vi "Centrifuge Module (Main).vi"(7 "Name of Parent Panel":string="Main.vi", 9 "New Center Coords":T1={"Horizontal"=470, "Vertical"=200}, 10 "Config":variant, 11 "Main UI Message Queue":refnum<queue>) -> ()   [LabVIEW 2018, in "Centrifuge Module.lvlib"]
doc: "This Continuous Measurement sample project is based on the Queued Message Handler template.\n\nThe Event Handling Loop generates messages based on user interface actions.\n\nThe Message Handling Loop processes messages generated by the Event Handling Loop, or by other messages. There are also Acquisition and Logging message handling loop subVIs, and a chart updating loop."
uses:
  Centrifuge Module.lvlib
  support/Message Queue/Message Cluster.ctl
  <vilib>/Utility/miscctls.llb/LVPoint32TypeDef.ctl
  controls/UI Data.ctl
  controls/UI State.ctl
  Centrifuge Module State Cluster.ctl
  Centrifuge Module Config Cluster.ctl
  Centrifuge Module Settings Cluster.ctl
  EPOS4/Controls/Device Selection.ctl
  EPOS4/Controls/EPOS Communication Settings.ctl
  Measure Instrument/State Enum.ctl
  Sequencing/Squence Update Cluster.ctl
  Centrifuge Module Display.ctl
  support/Message Queue/Enqueue Message (Single).vi
  support/User Event - Stop/User Event - Stop.lvlib
  support/Support Library.lvlib
  support/Message Queue/Message Queue.lvlib
  Measure Instrument/Centrifuge Module Engine.lvlib
  Measure Instrument/Feed Module Engine.lvlib
  Sequencing/Sequencing Library.lvlib
  Centrifuge Settings Dialog.vi
  support/Command Log VIs/Command Logging.lvlib
  EPOS4/EPOS4.lvlib
panel:
  out "Display Cluster":cluster{"User Name":string, "Speed":dbl} {"Speed" format="%#_5g"}
  out "H/W":dbl
  out "Original Height":u32
  out "Original Width":u32
  in  "Settings Button":bool
  out "Sequence Started":bool
  out "ScanCode":i16
  out "Ring":u16(ring)=2
  out "Log File path":path
  out "Status":string
  in  "Exit":bool
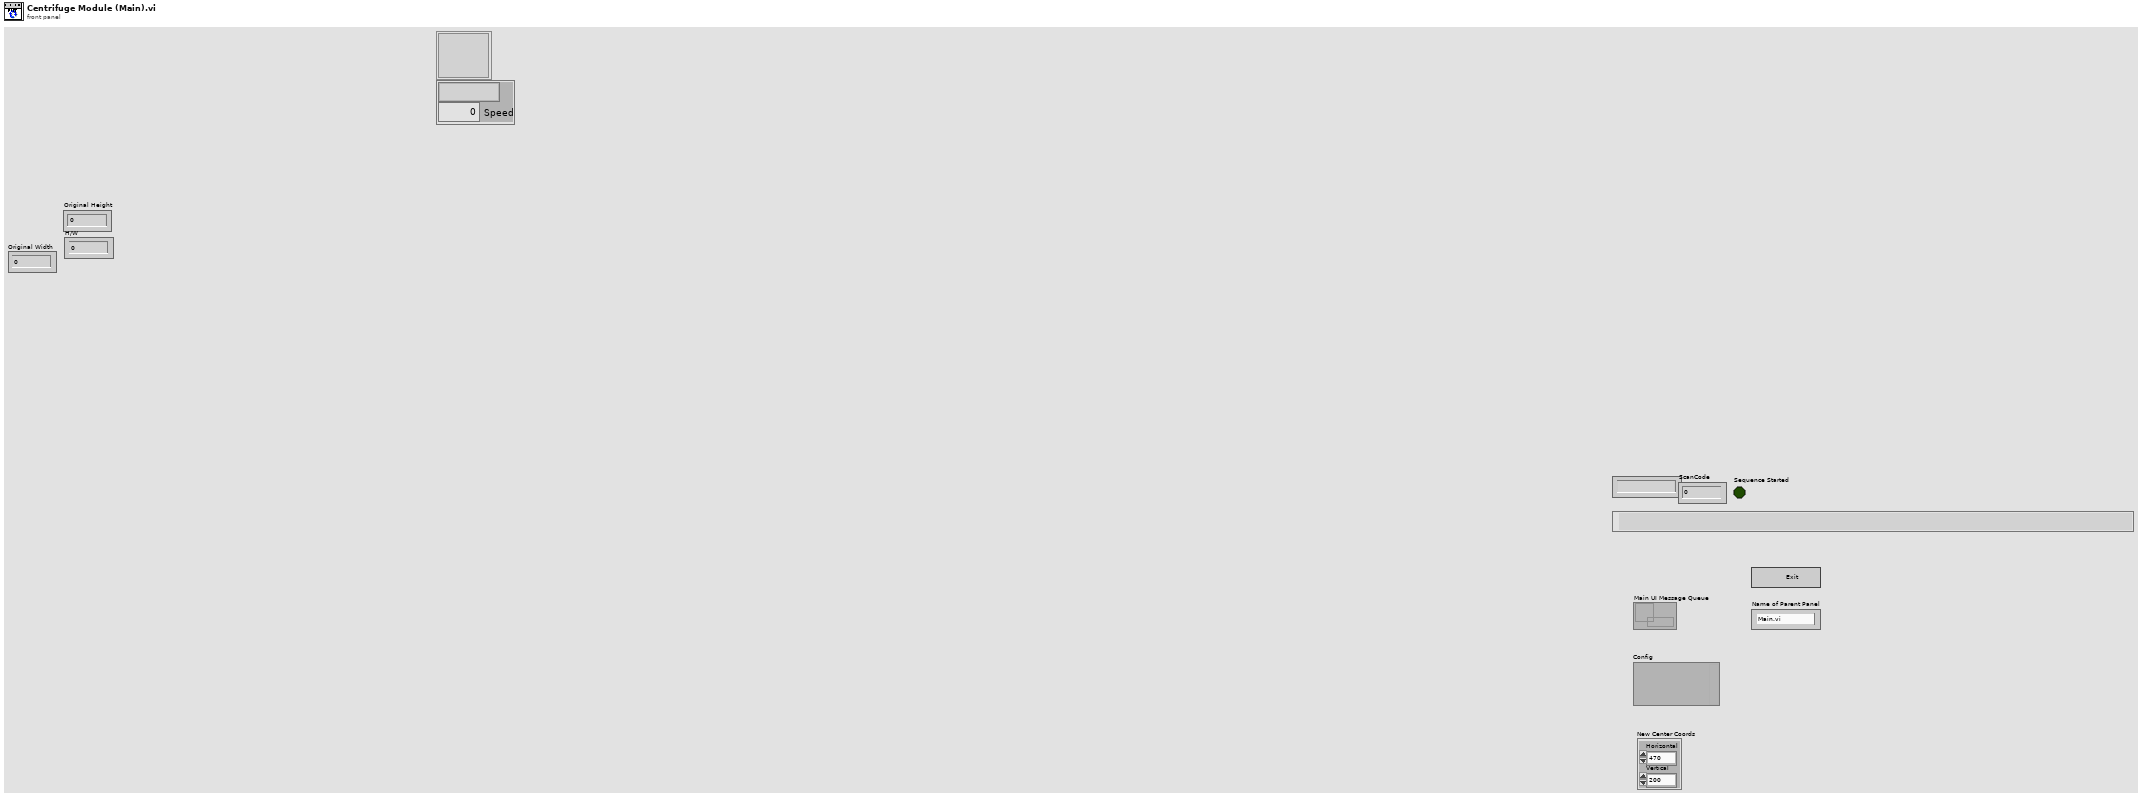
[diagram p1: front panel]
types:
  T1 = typedef "LVPoint32TypeDef.ctl" = cluster{"Horizontal":i32, "Vertical":i32}
  T2 = enum32{"Invalid", "Default", "Floating", "Floating/Auto-Hide", "Modal"}
  T3 = typedef "UI State.ctl" = enum16{"Idle", "Acquiring and Logging", "Waiting for Exit", "Waiting for Exit (Acq Stopped)", "Waiting for Exit (Log Stopped)", "Waiting for Stop", "Waiting for Stop (Acq Stopped)", "Waiting for Stop (Log Stopped)"}
  T4 = typedef "UI Data.ctl" = cluster{"Start Ref":refnum<vi>, "Trigger Ref":refnum<vi>, "Stop Ref":refnum<vi>, "Settings Ref":refnum<vi>, "Status Ref":refnum<vi>, "Exit Ref":refnum<vi>, "Data Ref":refnum<vi>}
  T5 = typedef "Centrifuge Module.lvlib/Centrifuge Module Config Cluster.ctl" = cluster{"GUID":string, "Drop Coords":T1, "Process Name":string, "User name":string, "Queue Name":string, "Settings":T6, "Load Count":i32}
  T6 = typedef "Centrifuge Module.lvlib/Centrifuge Module Settings Cluster.ctl" = cluster{"Cycle Period":dbl, "Manual Entry":dbl, "Output Device":T7, "EPOS4 Settings":T8}
  T7 = typedef "Device Selection.ctl" = enum16{"Default", "EPOS4"}
  T8 = typedef "EPOS4.lvlib/EPOS Communication Settings.ctl" = cluster{"VISA resource name":refnum<visa-resource-name>, "axis":cluster{"keyHandle":u32, "nodeId":u16}, "Simulated?":bool}
  T9 = typedef "Centrifuge Module.lvlib/Centrifuge Module State Cluster.ctl" = cluster{"Centrifuge Module Config":T5, "State":T10, "Start Time":timestamp, "Current Time":timestamp, "First Iteration":bool, "Data":cluster{"Centrifuge Speed":dbl}, "Process Name":string, "Centrifuge On?":bool}
  T10 = typedef "Feed Module.lvlib/Feed Module Engine.lvlib/State Enum.ctl" = enum16{"Measuring", "Idle", "Paused"}
  T11 = typedef "LVPointTypeDef.ctl" = cluster{"Horizontal":i16, "Vertical":i16}
  T12 = typedef "Centrifuge Module.lvlib/All Message Queues.ctl" = cluster{"Engine":refnum<queue>, "Centrifuge UI":refnum<queue>, "Centrifuge Engine":refnum<queue>, "Centrifuge Display":refnum<queue>}
  T13 = typedef "Sequencing Library.lvlib/Squence Update Cluster.ctl" = cluster{"Auto?":bool, "Manual Entry":dbl, "Setpoint":dbl}
  T14 = enum8{"Enabled", "Disabled", "Disabled and Grayed Out"}
  T15 = typedef "Centrifuge Module.lvlib/Centrifuge Module Display.ctl" = cluster{"Centrifuge On?":enum16{"Off", "On", "Not Initialized"}, "Cycle Period":dbl, "Current Centrifuge Speed":dbl, "Output":T7}
  T16 = typedef "LVRectTypeDef.ctl" = cluster{"Left":i16, "Top":i16, "Right":i16, "Bottom":i16}
  T17 = cluster{"Shift":bool, "Ctrl":bool, "Alt":bool, "Cmd":bool, "Opt":bool}
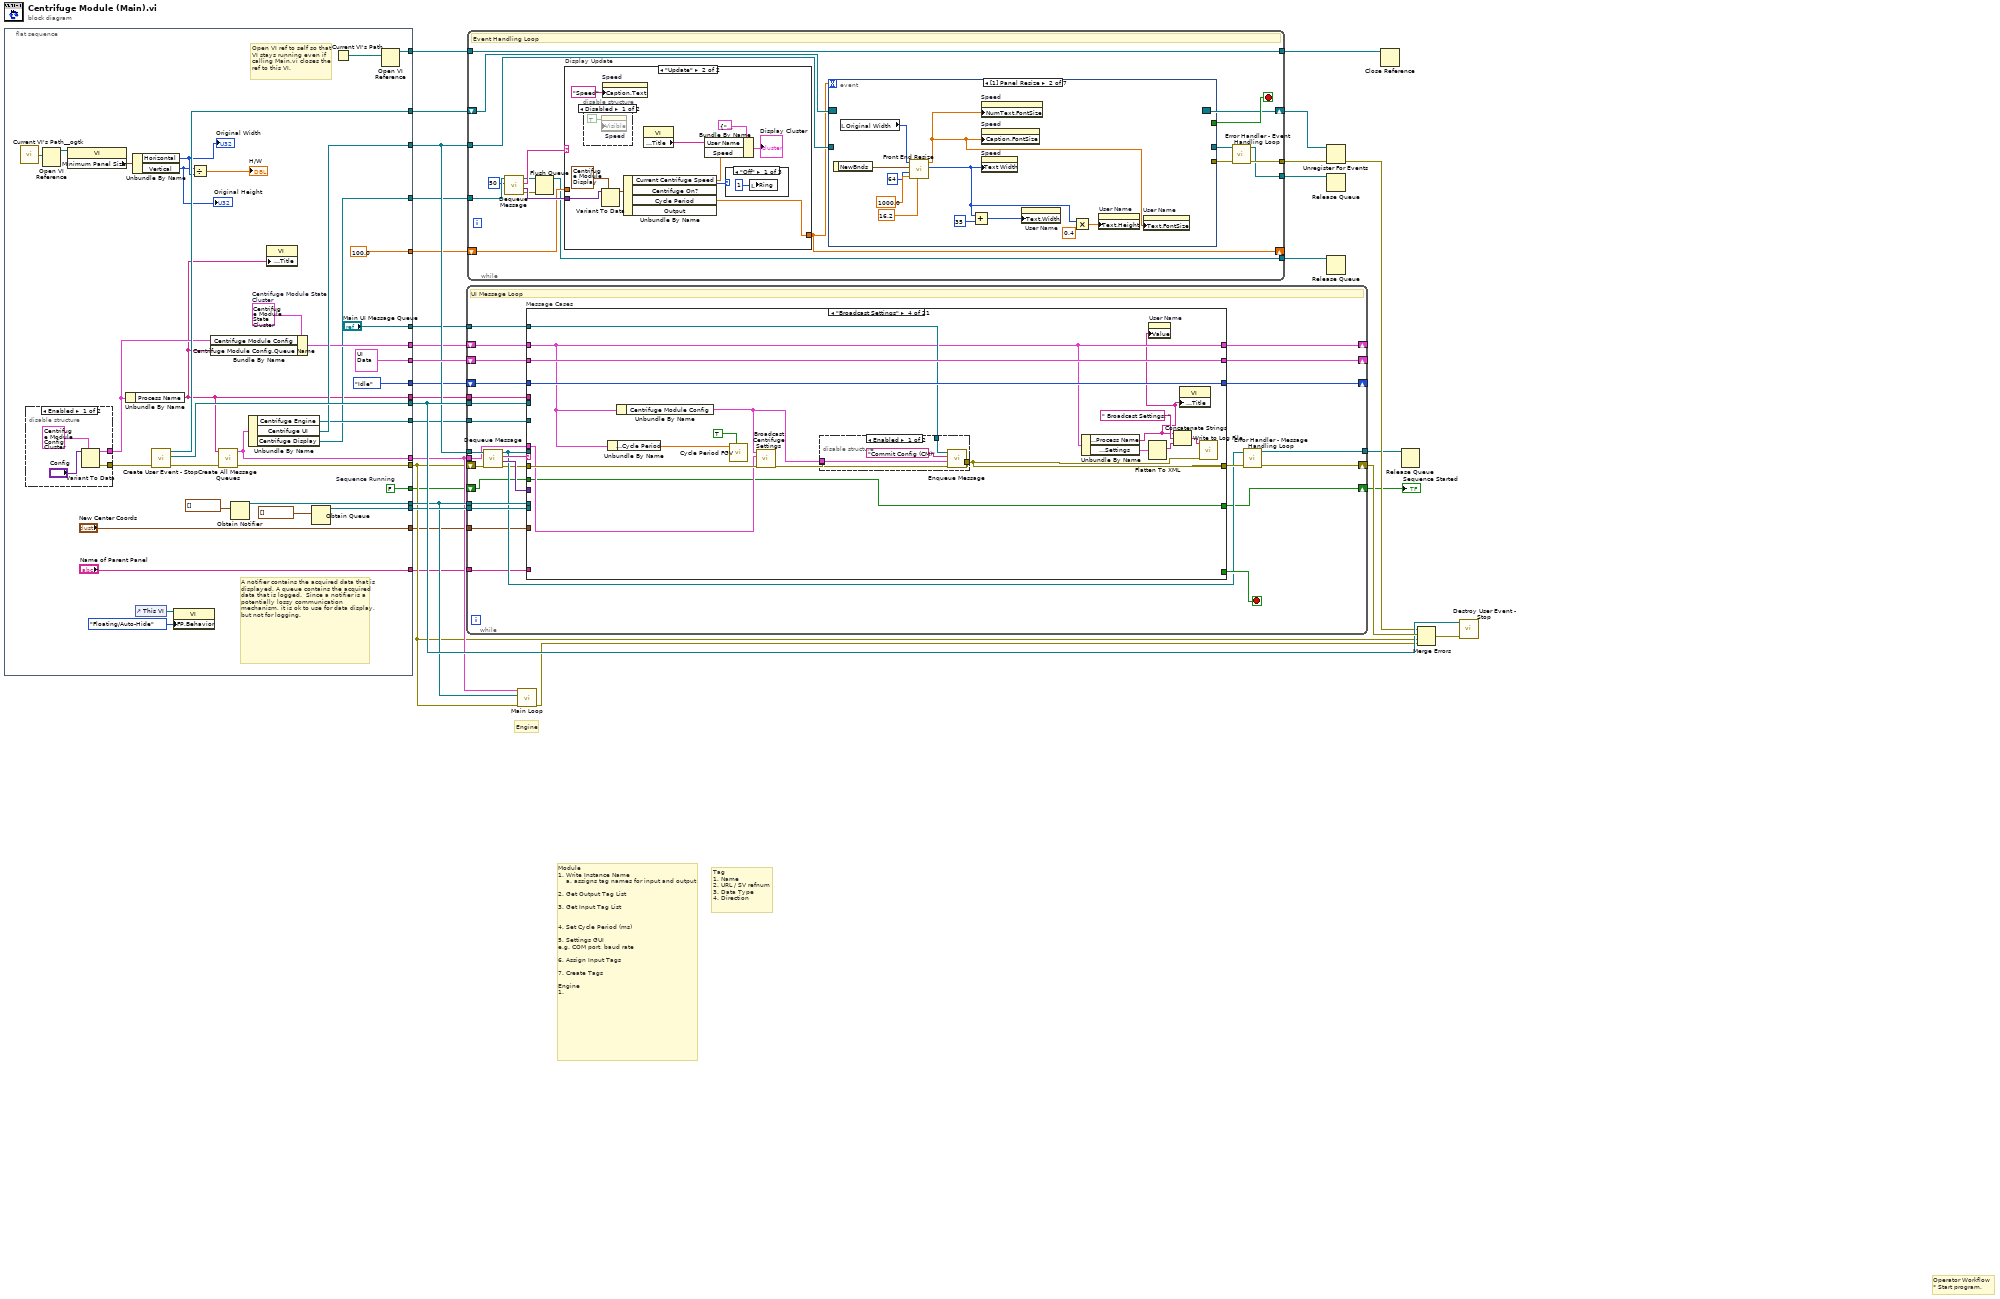
[diagram p0: block diagram]
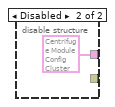
[diagram p2: hidden frame]
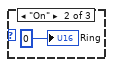
[diagram p5: hidden frame]
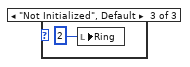
[diagram p6: hidden frame]
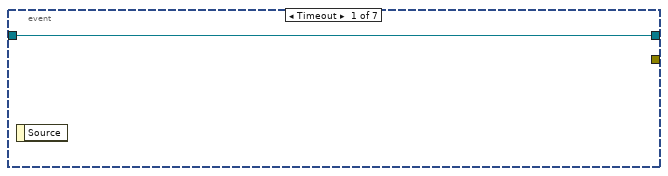
[diagram p7: hidden frame]
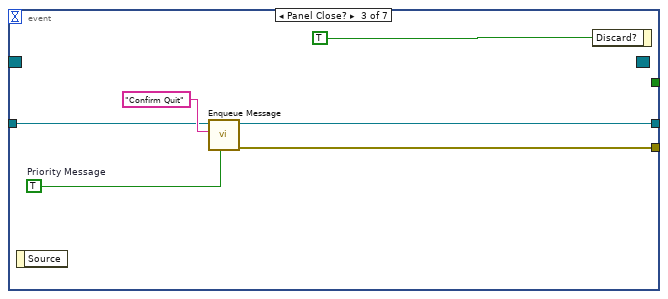
[diagram p8: hidden frame]
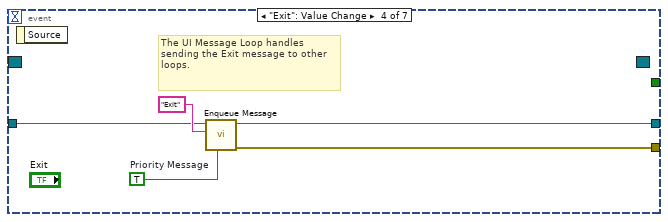
[diagram p9: hidden frame]
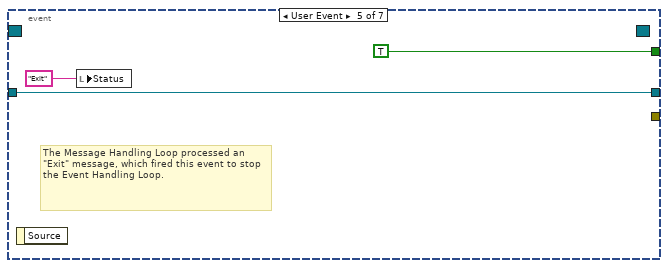
[diagram p10: hidden frame]
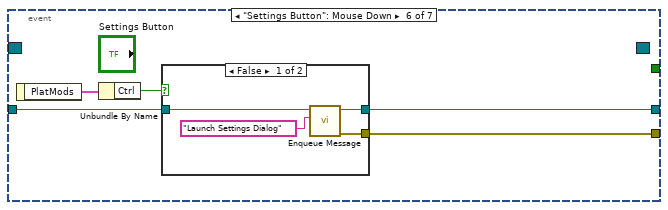
[diagram p11: hidden frame]
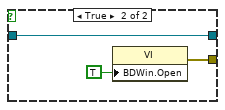
[diagram p12: hidden frame]
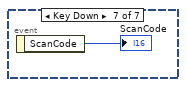
[diagram p13: hidden frame]
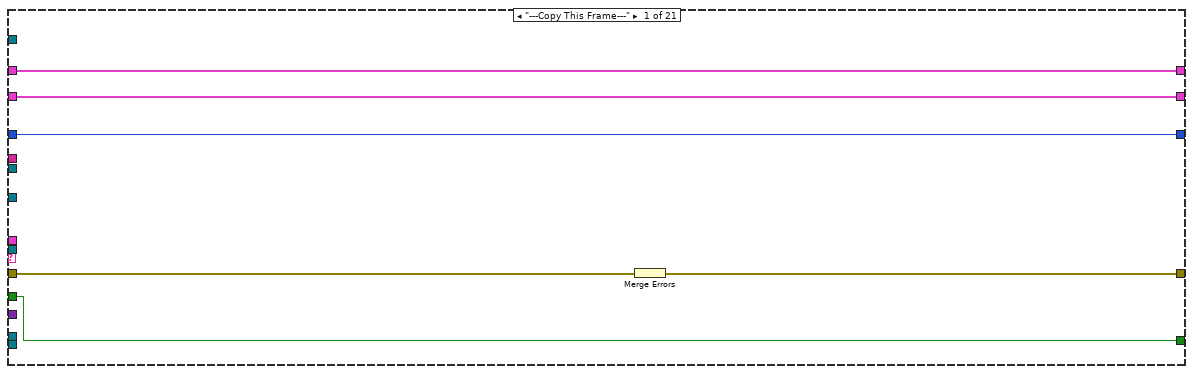
[diagram p14: hidden frame]
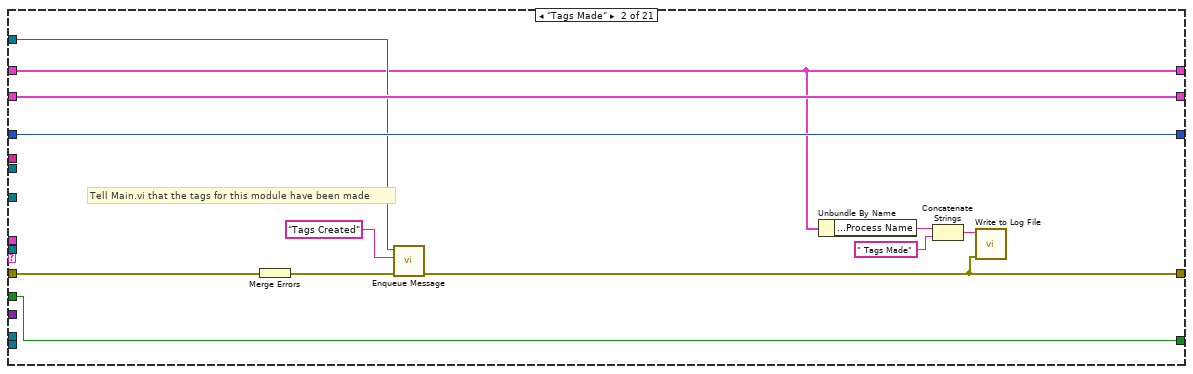
[diagram p15: hidden frame]
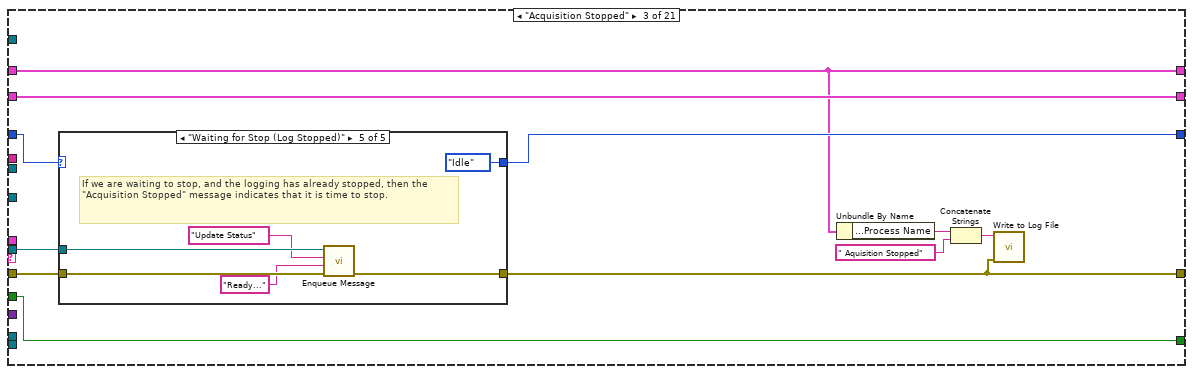
[diagram p16: hidden frame]
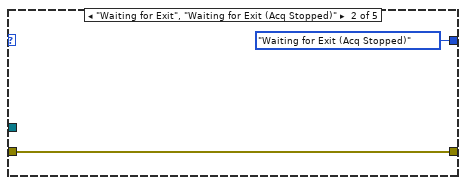
[diagram p18: hidden frame]
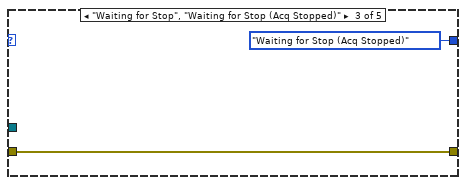
[diagram p19: hidden frame]
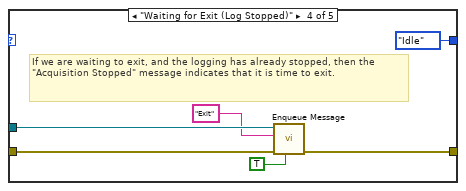
[diagram p20: hidden frame]
diagram:
  # "Engine"
  # "Operator Workflow\n* Start program."
  # "Module \n1. Write Instance Name\n    a. assigns tag names for input and output\n\n2. Get Output Tag List\n\n3. Get Input Tag List\n\n\n4. Set Cycle Period (ms)\n\n5. Settings GUI\ne.g. COM port, baud rate\n\n6. Assign Input Tags\n\n7. Create Tags\n\nEngine\n1."
  # "Tag\n1. Name\n2. URL / SV refnum\n3. Data Type\n4. Direction"
  n1 = flat-sequence {
    tunnel: [w64] -> w27
    tunnel: [w63] -> w26
    tunnel: [T4 {"Start Ref"=refnum, "Trigger Ref"=refnum, "Stop Ref"=refnum, "Settings Ref"=refnum, "Status Ref"=refnum, "Exit Ref"=refnum, "Data Ref"=refnum} ("Measurement UI Controls")] -> w23
    tunnel: [w61] -> w22
    tunnel: [UI_State."Idle" ("UI State")] -> w21
    tunnel: [w57] -> w20
    tunnel: [w56] -> w19
    tunnel: [w55] -> w17
    tunnel: [w54] -> w15
    tunnel: [w52] -> w14
    tunnel: ["Main UI Message Queue"] -> w13
    tunnel: [w47] -> w12
    tunnel: [w45] -> w11
    tunnel: [w44] -> w10
    tunnel: ["New Center Coords"] -> w9
    tunnel: ["Name of Parent Panel"] -> w8
    tunnel: [w41] -> w6
    tunnel: [w37] -> w5
    tunnel: [100.0 ("Cycle Period")] -> w4
    frame #0 {
      w41 = FALSE  # Sequence Running
      w48 = T9 {"Centrifuge Module Config"={"GUID"="", "Drop Coords"={"Horizontal"=0, "Vertical"=0}, "Process Name"="", "User name"="", "Queue Name"="", "Settings"={"Cycle Period"=500.0, "Manual Entry"=0.0, "Output Device"=enum."Default", "EPOS4 Settings"={"VISA resource name"="", "axis"={"keyHandle"=1, "nodeId"=1}, "Simulated?"=TRUE}}, "Load Count"=0}, "State"=enum."Idle", "Start Time"=timestamp(0 s since 1904-01-01), "Current Time"=timestamp(0 s since 1904-01-01), "First Iteration"=FALSE, "Data"={"Centrifuge Speed"=0.0}, "Process Name"="", "Centrifuge On?"=FALSE}  # Centrifuge Module State Cluster
      # "Open VI ref to self so that\nVI stays running even if\ncalling Main.vi closes the\nref to this VI."
      # "A notifier contains the acquired data that is displayed. A queue contains the acquired data that is logged.  Since a notifier is a potentially lossy communication mechanism, it is ok to use for data display, but not for logging."
      n2 = call <userlib>:"Current VI's Path__ogtk.vi"() -> ("Current VI's Path (+ Relative)"=w33:path)  [unwired: 1 in]
      n3 = disable-structure shown="Enabled" {
        disable-tunnel: [w68 _] -> w51
        disable-tunnel: [w67 T5 {"GUID"="", "Drop Coords"={"Horizontal"=0, "Vertical"=0}, "Process Name"="", "User name"="", "Queue Name"="", "Settings"={"Cycle Period"=500.0, "Manual Entry"=0.0, "Output Device"=enum."Default", "EPOS4 Settings"={"VISA resource name"="", "axis"={"keyHandle"=1, "nodeId"=1}, "Simulated?"=TRUE}}, "Load Count"=0} ("Feed Module Config")] -> w50
        frame Enabled {
          n4 = Variant To Data(type=T5 {"GUID"="", "Drop Coords"={"Horizontal"=0, "Vertical"=0}, "Process Name"="", "User name"="", "Queue Name"="", "Settings"={"Cycle Period"=500.0, "Manual Entry"=0.0, "Output Device"=enum."Default", "EPOS4 Settings"={"VISA resource name"="", "axis"={"keyHandle"=1, "nodeId"=1}, "Simulated?"=TRUE}}, "Load Count"=0} ("Feed Module Config"), Variant="Config") -> (data=w67:T5, error out=w68:errorcluster)  [unwired: 1 in]
        }
        frame Disabled {
        }
      }
      n5 = Open VI Reference(vi path=w33) -> (vi reference=w34:refnum<vi>)  [unwired: 5 in, 1 out]
      n6 = property class="VI"(reference=w34) -> ("Minimum Panel Size"=w35:T11)  [unwired: 1 in, 2 out]
      n7 = Unbundle By Name(w50) -> ("Process Name"=w37:string)
      n8 = Unbundle By Name(w35) -> ("Horizontal"=w36:i16, "Vertical"=w31:i16)
      "Original Width" <- w36
      "Original Height" <- w31
      n9 = control-ref of="This VI"() -> (w39:refnum<vi>)
      n10 = call "Create User Event - Stop.vi"("error in (no error)"=w51) -> ("error out"=w46:errorcluster, "User Event - Stop"=w63:refnum<user-event>, "Stop Event Registration Refnum"=w64:refnum<event-registration>)  [unwired: 8 in]
      n11 = property class="VI"(reference=w39, "FP.Behavior"=T2."Floating/Auto-Hide" ("Front Panel Window:Behavior")) -> ()  [unwired: 1 in, 2 out]
      n12 = Divide(x=w31, y=w36) -> (x/y=→"H/W":dbl)
      n13 = Bundle By Name(cluster=w48, "Centrifuge Module Config"=w50, "Centrifuge Module Config.Queue Name"=w37) -> (w52:T9)
      n14 = call "Create All Message Queues.vi"("error in (no error)"=w46, "Process Name"=w37) -> ("error out"=w44:errorcluster, "Message Queues"=w45:T12)  [unwired: 8 in]
      n15 = Obtain Notifier(notification data type=waveform(dbl)[] []) -> (notifier out=w55:refnum<notifier>)  [unwired: 3 in, 2 out]
      n16 = Unbundle By Name(w45) -> ("Centrifuge Engine"=w57:refnum<queue>, "Centrifuge UI"=w61:refnum<queue>, "Centrifuge Display"=w47:refnum<queue>)
      n17 = property class="VI"("Front Panel.Title"=w37) -> ()  [unwired: 2 in, 2 out]
      n18 = Obtain Queue(element data type=waveform(dbl)[] []) -> (queue out=w56:refnum<queue>)  [unwired: 4 in, 2 out]
      n19 = Current VI's Path() -> (path=w53:path)
      n20 = Open VI Reference(vi path=w53) -> (vi reference=w54:refnum<vi>)  [unwired: 5 in, 1 out]
    }
  }
  n21 = while {
    tunnel: w22 -> [w91]
    tunnel: w26 -> [w95]
    shift-right: [w85] -> w30
    shift-left: w10 -> [w94]
    shift-right: [w78] -> _
    shift-left: w14 -> [w71]
    shift-right: [w89] -> _
    shift-left: w23 -> [w90]
    tunnel: w17 -> [w88]
    tunnel: w19 -> [w87]
    shift-right: [w82] -> _
    shift-left: w21 -> [w83]
    tunnel: w20 -> [w81]
    tunnel: w13 -> [w79]
    tunnel: w11 -> [w77]
    tunnel: w5 -> [w76]
    tunnel: w9 -> [w75]
    tunnel: w8 -> [w74]
    shift-right: [w73] -> w7
    shift-left: w6 -> [w72]
    tunnel: [w70] -> w1
    stop <- w96 stop-if-true
    # "UI Message Loop"
    n22 = call "Dequeue Message.vi"("error in (no error)"=w94, "Message Queue"=w91) -> ("error out"=w80:errorcluster, "Message Data"=w92:variant, "Message"=w93:string, "dup Message Queue"=w84:refnum<queue>)  [unwired: 6 in]
    n23 = case "Message Cases" shown="\"Broadcast Settings\"" w93 {
      selector: w93 -> [_ _ _ _ _ _ _ _ _ _ _ _ _ _ _ _ _ _ _ _ w559]
      tunnel: w84 -> [_ _ w121 _ w176 w199 _ w264 w279 w307 _ w343 w363 w379 w415 w454 _ _ w514 _ _]
      tunnel: w80 -> [w102 w114 w122 w156 w175 w198 w231 w245 w283 w311 w327 w338 w362 w380 w413 w453 w474 w489 w516 w550 _]
      tunnel: [w101 w105 w117 w151 w171 w196 w232 w239 w268 w287 w327 w330 w353 w374 w407 w441 w482 w491 w508 w551 w558] -> w86
      tunnel: [_ _ _ _ _ _ _ _ _ TRUE _ _ _ _ _ _ _ _ _ _ _] -> w96
      tunnel: w92 -> [_ _ _ _ w177 _ w234 _ w282 w295 _ _ _ _ _ _ _ _ _ w549 _]
      tunnel: w95 -> [_ _ _ _ _ _ _ _ _ w310 _ _ _ _ _ _ _ _ _ _ _]
      tunnel: w71 -> [w98 w104 w116 w148 w169 w195 w229 w243 w270 w286 w318 w329 w352 w375 w405 w449 w475 w490 w518 w540 w564]
      tunnel: w90 -> [w100 w113 w125 w160 w178 w201 w236 w261 w284 w308 w326 w339 w365 w383 w410 w450 w481 w500 w534 w546 w569]
      tunnel: [w100 w113 w125 w160 w178 w201 w236 w261 w284 w308 w325 w339 w365 w383 w410 w450 w481 w500 w534 w546 w569] -> w89
      tunnel: w88 -> [_ _ _ _ _ _ _ _ _ w306 _ _ _ _ _ _ _ _ _ _ _]
      tunnel: w87 -> [_ _ _ _ _ _ _ _ _ w302 _ _ _ _ _ _ _ _ _ _ _]
      tunnel: w83 -> [w99 w112 w124 w159 w179 w200 w230 w250 w274 _ _ _ w364 w382 _ _ _ _ w523 w541 w568]
      tunnel: [w99 w112 w123 w159 w179 w197 w230 w251 w274 UI_State."Idle" ("UI State") UI_State."Idle" ("UI State") UI_State."Idle" ("UI State") w364 w381 UI_State."Acquiring and Logging" ("UI State") UI_State."Acquiring and Logging" ("UI State") UI_State."Acquiring and Logging" ("UI State") UI_State."Acquiring and Logging" ("UI State") w524 w541 w568] -> w82
      tunnel: w81 -> [_ _ _ _ _ _ _ w249 _ w294 _ _ _ _ _ _ w479 w498 w522 _ _]
      tunnel: w79 -> [_ w109 _ w155 _ _ _ _ _ w296 _ _ _ _ _ _ _ _ _ _ _]
      tunnel: [w98 w104 w116 w148 w168 w195 w229 w238 w270 w286 w318 w329 w354 w375 w404 w440 w475 w490 w507 w540 w564] -> w78
      tunnel: w77 -> [_ _ _ w153 _ _ _ _ _ _ _ _ w361 _ _ _ _ _ _ _ _]
      tunnel: w76 -> [_ _ _ _ _ _ _ _ _ _ _ w334 _ _ _ _ _ _ _ _ _]
      tunnel: w75 -> [_ _ _ _ _ _ _ _ _ _ _ w336 _ _ _ _ _ _ _ _ _]
      tunnel: w74 -> [_ _ _ _ _ _ _ _ _ _ _ w335 _ _ _ _ _ _ _ _ _]
      tunnel: [w97 w103 w115 w145 w167 w194 w228 w237 w267 w285 w317 w328 w350 w373 w402 w447 w473 w488 w506 w539 w557] -> w73
      tunnel: w72 -> [w97 w103 w115 w145 w167 w194 w228 w237 w267 w285 w317 w328 w350 w373 w402 w445 w473 w488 w506 w539 w557]
      frame "---Copy This Frame---" {
        # "Duplicate this frame when creating new messages.  Change this comment in the duplicated frame to describe this message."
        n24 = Merge Errors(w102) -> (w101:errorcluster)
      }
      frame "Tags Made" {
        # "Tell Main.vi that the tags for this module have been made"
        # "Duplicate this frame when creating new messages.  Change this comment in the duplicated frame to describe this message."
        n25 = Merge Errors(w114) -> (w110:errorcluster)
        n26 = call-poly "Enqueue Message.vi"("error in (no error)"=w110, "Message"="Tags Created", "Message Queue"=w109) -> ("error out"=w105:errorcluster)  [unwired: 7 in, 1 out]
        n27 = Unbundle By Name(w104) -> ("Centrifuge Module Config.Process Name"=w108:string)
        n28 = Concatenate Strings(w108, " Tags Made" ("text")) -> (w106:string)
        n29 = call "Write to Log File.vi"("error in"=w105, "text"=w106) -> ()  [unwired: 9 in, 1 out]
      }
      frame "Acquisition Stopped" {
        # "Logic for determining what action to take when the acquisition has stopped."
        n30 = case shown="\"Waiting for Stop (Log Stopped)\"" w124 {
          selector: w124 -> [w127 _ _ _ _]
          tunnel: [w127 UI_State."Waiting for Exit (Acq Stopped)" ("UI State") UI_State."Waiting for Stop (Acq Stopped)" ("UI State") UI_State."Idle" ("UI State") UI_State."Idle" ("UI State")] -> w123
          tunnel: w122 -> [w126 w128 w130 w136 w142]
          tunnel: [w126 w128 w130 w135 w141] -> w117
          tunnel: w121 -> [_ _ _ w134 w140]
          frame Default {
          }
          frame "Waiting for Exit", "Waiting for Exit (Acq Stopped)" {
          }
          frame "Waiting for Stop", "Waiting for Stop (Acq Stopped)" {
          }
          frame "Waiting for Exit (Log Stopped)" {
            # "If we are waiting to exit, and the logging has already stopped, then the \"Acquisition Stopped\" message indicates that it is time to exit."
            n31 = call-poly "Enqueue Message.vi"("Priority Message? (F)"=TRUE, "error in (no error)"=w136, "Message"="Exit", "Message Queue"=w134) -> ("error out"=w135:errorcluster)  [unwired: 6 in, 1 out]
          }
          frame "Waiting for Stop (Log Stopped)" {
            # "If we are waiting to stop, and the logging has already stopped, then the \"Acquisition Stopped\" message indicates that it is time to stop."
            n32 = call-poly "Enqueue Message.vi"("error in (no error)"=w142, "Message Data"="Ready..." ("Message"), "Message"="Update Status", "Message Queue"=w140) -> ("error out"=w141:errorcluster)  [unwired: 6 in, 1 out]
          }
        }
        n33 = Unbundle By Name(w116) -> ("Centrifuge Module Config.Process Name"=w120:string)
        n34 = Concatenate Strings(w120, " Aquisition Stopped" ("text")) -> (w118:string)
        n35 = call "Write to Log File.vi"("error in"=w117, "text"=w118) -> ()  [unwired: 9 in, 1 out]
      }
      frame "Broadcast Settings" {
        # "Send the 'Update Settings' message to the Logging and Acquisition message loops."
        n36 = Unbundle By Name(w148) -> ("Centrifuge Module Config.Settings.Cycle Period"=w157:dbl)
        n37 = Unbundle By Name(w148) -> ("Centrifuge Module Config"=w152:T5)
        n38 = call "Cycle Period FGV.vi"("Write"=TRUE, "Cycle Period In (ms)"=w157) -> ()  [unwired: 8 in, 2 out]
        n39 = call "Broadcast Centrifuge Settings.vi"("error in (no error)"=w156, "Message Queues"=w153, "Pump Module Config"=w152) -> ("error out"=w154:errorcluster)  [unwired: 8 in]
        n40 = disable-structure shown="Enabled" {
          disable-tunnel: w155 -> [w165 _]
          disable-tunnel: w154 -> [w164 w166]
          disable-tunnel: w152 -> [w162 _]
          disable-tunnel: [w161 w166] -> w151
          frame Enabled {
            n41 = call-poly "Enqueue Message.vi"("error in (no error)"=w164, "Message Data"=w162, "Message"="Commit Config (CM)", "Message Queue"=w165) -> ("error out"=w161:errorcluster)  [unwired: 6 in, 1 out]
          }
          frame Disabled {
          }
        }
        n42 = Unbundle By Name(w148) -> ("Centrifuge Module Config.Process Name"=w144:string, "Centrifuge Module Config.Settings"=w146:T6)
        n43 = Flatten To XML(anything=w146) -> (xml string=w147:string)
        n44 = property on="User Name" class="Str"("Value"=w144) -> ()  [unwired: 2 in, 2 out]
        n45 = Concatenate Strings(w144, " Broadcast Settings: " ("text"), w147) -> (w149:string)
        n46 = property class="VI"("Front Panel.Title"=w144) -> ()  [unwired: 2 in, 2 out]
        n47 = call "Write to Log File.vi"("error in"=w151, "text"=w149) -> ()  [unwired: 9 in, 1 out]
      }
      frame "Sequence Update" {
        n48 = in-place {
          in-place-border: w177 -> [w190]
          in-place-border: w175 -> [w189]
          in-place-border: [w188] -> w174
          n49 = in-place-cluster #1(w169) -> ("Centrifuge Module Config"=w186:T5)
          n50 = Variant To Data(error in=w189, type=T13 {"Auto?"=TRUE, "Manual Entry"=0.0, "Setpoint"=0.0} ("Cluster"), Variant=w190) -> (data=w192:T13, error out=w188:errorcluster)
          n51 = Unbundle By Name(w192) -> ("Manual Entry"=w191:dbl)
          n52 = Bundle By Name(cluster=w186, "Settings.Manual Entry"=w191) -> (w187:T5)
          n53 = in-place-cluster #1("Centrifuge Module Config"=w187) -> (w168:T9)
        }
        n54 = disable-structure shown="Disabled" {
          disable-tunnel: [w184 w185] -> w180
          disable-tunnel: w176 -> [w182 _]
          disable-tunnel: w174 -> [w181 w185]
          frame Disabled {
            n55 = call-poly "Enqueue Message.vi"("error in (no error)"=w181, "Message"="Broadcast Settings", "Message Queue"=w182) -> ("error out"=w184:errorcluster)  [unwired: 7 in, 1 out]
          }
          frame Enabled {
          }
        }
        n56 = Merge Errors(w180) -> (w171:errorcluster)
        n57 = Unbundle By Name(w168) -> ("Centrifuge Module Config.Process Name"=w173:string)
        n58 = Concatenate Strings(w173, "Sequence Update" ("text")) -> (w170:string)
        n59 = call "Write to Log File.vi"("error in"=w171, "text"=w170) -> ()  [unwired: 9 in, 1 out]
      }
      frame "Confirm Quit" {
        # "Confirm Quit - Message that can confirm whether or not the user wants to exit the application."
        n60 = case shown="\"Acquiring and Logging\"" w200 {
          tunnel: w199 -> [w206 w213]
          tunnel: w198 -> [w205 w211]
          tunnel: [w202 w210] -> w196
          tunnel: [UI_State."Idle" ("UI State") w209] -> w197
          tunnel: w195 -> [_ w208]
          frame Default {
            # "If 'Confirm Quit' comes in while the system is idle, there is no need for a confirmation message."
            n61 = call-poly "Enqueue Message.vi"("Priority Message? (F)"=TRUE, "error in (no error)"=w205, "Message"="Exit", "Message Queue"=w206) -> ("error out"=w202:errorcluster)  [unwired: 6 in, 1 out]
          }
          frame "Acquiring and Logging" {
            n62 = Two Button Dialog(message="Are you sure you want to quit while the acquisition is running?" ("Confirm Quit Message"), 1:"No" ("No"), 2:"Yes" ("Yes")) -> (T button?=w212:bool)
            n63 = case shown="True" w212 {
              tunnel: w213 -> [_ w227]
              tunnel: w211 -> [w217 w226]
              tunnel: [w217 w219] -> w210
              tunnel: [UI_State."Acquiring and Logging" ("UI State") UI_State."Waiting for Exit" ("UI State")] -> w209
              tunnel: w208 -> [_ w220]
              frame False {
                # "User did not want to quit."
              }
              frame True {
                n64 = call-poly "Enqueue Message.vi"("error in (no error)"=w226, "Message"="Stop", "Message Queue"=w227) -> ("error out"=w219:errorcluster)  [unwired: 7 in, 1 out]
                n65 = Unbundle By Name(w220) -> ("Centrifuge Module Config.Process Name"=w222:string)
                n66 = Concatenate Strings(w222, " Quit" ("text")) -> (w223:string)
                n67 = call "Write to Log File.vi"("error in"=w219, "text"=w223) -> ()  [unwired: 9 in, 1 out]
              }
            }
          }
        }
      }
      frame "Display Log File Path" {
        n68 = Variant To Data(error in=w231, type=path "", Variant=w234) -> (data=→"Log File path":path, error out=w232:errorcluster)
      }
      frame "E-Stop" {
        # "Pause the pump when there is an E-STOP"
        # "Message Acquisition and Logging loops to stop"
        # "Enable: Start, Exit, Settings\nDisable: Stop"
        # "Stop the pumps."
        n69 = Unbundle By Name(w261) -> ("Trigger Ref"=w252:refnum<vi>, "Stop Ref"=w253:refnum<vi>, "Start Ref"=w256:refnum<vi>, "Exit Ref"=w255:refnum<vi>, "Settings Ref"=w254:refnum<vi>)
        n70 = call-poly "Enqueue Message.vi"("error in (no error)"=w245, "Message Data"="Ready..." ("Ready..."), "Message"="Update Status", "Message Queue"=w264) -> ("error out"=w247:errorcluster)  [unwired: 6 in, 1 out]
        n71 = Build Array(w256, w255, w254) -> (w259:refnum<vi>[])
        n72 = Build Array(w252, w253) -> (w258:refnum<vi>[])
        n73 = call-poly "Enqueue Message.vi"("error in (no error)"=w247, "Message"="Pause", "Message Queue"=w249) -> ("error out"=w246:errorcluster)  [unwired: 7 in, 1 out]
        n74 = call "Set Enable State on Multiple Controls.vi"("Enable?"=FALSE, "Controls"=w258) -> ()  [unwired: 10 in]
        n75 = call "Set Enable State on Multiple Controls.vi"("Enable?"=TRUE, "Controls"=w259) -> ()  [unwired: 10 in]
        n76 = case shown="Default" w250 {
          selector: w250 -> [_ w266]
          tunnel: [UI_State."Waiting for Stop" ("UI State") w266] -> w251
          frame Default {
          }
          frame "Waiting for Exit" {
          }
        }
        n77 = Merge Errors(w246) -> (w239:errorcluster)
        n78 = Bundle By Name(cluster=w243, "State"=State_Enum."Idle") -> (w238:T9)
        n79 = Unbundle By Name(w238) -> ("Centrifuge Module Config.Process Name"=w242:string)
        n80 = Concatenate Strings(w242, " E-STOP" ("text")) -> (w240:string)
        n81 = call "Write to Log File.vi"("error in"=w239, "text"=w240) -> ()  [unwired: 9 in, 1 out]
      }
      frame "Error" {
        # "Error - Check the error message data and respond accordingly. This message is sent by the \"Error Handler\" VIs at the end of each loop in this application."
        n82 = Variant To Data(error in=w283, type=errorcluster {"status"=FALSE, "code"=0, "source"=""} ("error out"), Variant=w282) -> (data=w280:errorcluster, error out=w276:errorcluster)
        n83 = call <vilib>:"General Error Handler.vi"("error in (no error)"=w280) -> ("message"=w269:string)  [unwired: 10 in, 4 out]
        n84 = call-poly "Enqueue Message.vi"("Priority Message? (F)"=TRUE, "Message"="Exit", "Message Queue"=w279) -> ("error out"=w275:errorcluster)  [unwired: 7 in, 1 out]
        n85 = Merge Errors(w275, w276) -> (w268:errorcluster)
        n86 = Unbundle By Name(w270) -> ("Centrifuge Module Config.Process Name"=w273:string)
        n87 = Concatenate Strings(w273, " Error: " ("text"), w269) -> (w271:string)
        n88 = call "Write to Log File.vi"("error in"=w268, "text"=w271) -> ()  [unwired: 9 in, 1 out]
      }
      frame "Exit" {
        w299 = TRUE  # Delete Module?
        # "Don't check the error outs. The acquisition and logging queues may have already been released."
        # "Close references owned by the Main VI."
        # "Stop the VI"
        # "Exit - Fire the User Event to stop the Event Handling Loop.  Also send Exit messages to the Acquisition and Logging loops."
        n89 = Release Queue(queue=w307, error in (no error)=w311) -> (error out=w305:errorcluster)  [unwired: 1 in, 2 out]
        n90 = call "Fire User Event - Stop.vi"("User Event - Stop"=w310) -> ("error out"=w309:errorcluster)  [unwired: 10 in]
        n91 = Release Notifier(notifier=w306, error in (no error)=w305) -> (error out=w304:errorcluster)  [unwired: 1 in, 2 out]
        n92 = Release Queue(queue=w302, error in (no error)=w304) -> (error out=w303:errorcluster)  [unwired: 1 in, 2 out]
        n93 = call-poly "Enqueue Message.vi"("Message"="Stop", "Message Queue"=w294) -> ("dup Message Queue"=w292:refnum<queue>)  [unwired: 8 in, 1 out]
        n94 = Variant To Data(type=w299, Variant=w295) -> (data=w298:bool, error out=w300:errorcluster)  [unwired: 1 in]
        n95 = Select(t=w299, s=w300, f=w298) -> (s? t:f=w297:bool)
        n96 = call-poly "Enqueue Message.vi"("Message"="Exit", "Message Queue"=w292) -> ()  [unwired: 8 in, 2 out]
        n97 = case "Don't enqueue Delete Module if opening campaign because it\nwill already have been deleted and new config loaded and we create\na race condition." shown="True" w297 {
          tunnel: w296 -> [_ w315]
          tunnel: w286 -> [_ w314]
          frame False {
          }
          frame True {
            n98 = Unbundle By Name(w314) -> ("Centrifuge Module Config.GUID"=w313:string)
            n99 = call-poly "Enqueue Message.vi"("Message Data"=w313, "Message"="Delete Module", "Message Queue"=w315) -> ()  [unwired: 7 in, 2 out]
          }
        }
        n100 = Merge Errors(w309, w303) -> (w287:errorcluster)
        n101 = Unbundle By Name(w286) -> ("Centrifuge Module Config.Process Name"=w290:string)
        n102 = Concatenate Strings(w290, " Exit" ("text")) -> (w288:string)
        n103 = call "Write to Log File.vi"("error in"=w287, "text"=w288) -> ()  [unwired: 9 in, 1 out]
      }
      frame "Init UI Refs" {
        # "Enable: Start, Exit, Settings\nDisable: Stop"
        # "Init UI Refs - Store control references for UI controls.  Also enable/disable controls appropriately."
        n104 = property class="VI"("Front Panel.Closeable"=TRUE ("Front Panel Window:Closeable")) -> ()  [unwired: 2 in, 2 out]
        n105 = control-ref of="Status"() -> (w323:refnum<vi>)
        n106 = control-ref of="Exit"() -> (w320:refnum<vi>)
        n107 = Bundle By Name(cluster=w326, "Status Ref"=w323, "Exit Ref"=w320) -> (w325:T4)
        n108 = Build Array(w320) -> (w322:refnum<vi>[])
        n109 = call "Set Enable State on Multiple Controls.vi"("Enable?"=TRUE, "Controls"=w322) -> ()  [unwired: 10 in]
      }
      frame "Initialize" {
        # "Initialize - Get configuration settings, then message the UI to initialize, and broadcast the settings to the other message loops."
        n110 = property class="VI" props=["FP.State"]() -> (reference out=w337:refnum<vi>)  [unwired: 2 in, 2 out]
        n111 = call-poly "Enqueue Message.vi"("error in (no error)"=w338, "Message"="Init UI Refs", "Message Queue"=w343) -> ("error out"=w341:errorcluster, "dup Message Queue"=w342:refnum<queue>)  [unwired: 7 in]
        n112 = call "Make Child and Move.vi"("Process Name"=w334, "Name of Parent Panel"=w335, "New Center Coords"=w336, "VI in"=w337) -> ()  [unwired: 8 in]
        n113 = call-poly "Enqueue Message.vi"("error in (no error)"=w341, "Message"="Broadcast Settings", "Message Queue"=w342) -> ("error out"=w349:errorcluster, "dup Message Queue"=w348:refnum<queue>)  [unwired: 7 in]
        n114 = call-poly "Enqueue Message.vi"("error in (no error)"=w349, "Message Data"="Ready..." ("Ready..."), "Message"="Update Status", "Message Queue"=w348) -> ("error out"=w330:errorcluster)  [unwired: 6 in, 1 out]
        n115 = Unbundle By Name(w329) -> ("Centrifuge Module Config.Process Name"=w333:string)
        n116 = Concatenate Strings(w333, " Initialize" ("text")) -> (w331:string)
        n117 = call "Write to Log File.vi"("error in"=w330, "text"=w331) -> ()  [unwired: 9 in, 1 out]
      }
      frame "Launch Settings Dialog" {
        # "Keep track of the number of times it has opened"
        # "Launch the Settings Dialog when the user clicks the 'Settings' button."
        n118 = in-place {
          n119 = in-place-cluster #2(w352) -> ("Centrifuge Module Config.Load Count"=w367:i32)
          n120 = Increment(x=w367) -> (x+1=w366:i32)
          n121 = in-place-cluster #2("Centrifuge Module Config.Load Count"=w366) -> (w351:T9)
        }
        n122 = call-by-ref "?"("error in (no error)"=w362, "Message Queues"=w361, "Pump Module State Cluster In"=w351) -> ("error out"=w359:errorcluster, "Cancelled?"=w358:bool, "Centrifuge Module Config Out"=w360:T5)  [unwired: 7 in, 3 out]
        n123 = case shown="True" w358 {
          tunnel: [w368 w372] -> w353
          tunnel: w363 -> [_ w371]
          tunnel: w359 -> [w368 w369]
          frame False {
          }
          frame True {
            # "Send out the settings"
            n124 = call-poly "Enqueue Message.vi"("error in (no error)"=w369, "Message"="Broadcast Settings", "Message Queue"=w371) -> ("error out"=w372:errorcluster)  [unwired: 7 in, 1 out]
          }
        }
        n125 = Bundle By Name(cluster=w352, "Centrifuge Module Config"=w360) -> (w354:T9)
        n126 = Unbundle By Name(w354) -> ("Centrifuge Module Config.Process Name"=w357:string)
        n127 = Concatenate Strings(w357, " Setting Dialog Launched" ("text")) -> (w355:string)
        n128 = call "Write to Log File.vi"("error in"=w353, "text"=w355) -> ()  [unwired: 9 in, 1 out]
      }
      frame "Logging Stopped" {
        # "Logic for determining what action to take when the logging has stopped."
        n129 = case shown="\"Waiting for Exit (Acq Stopped)\"" w382 {
          selector: w382 -> [w385 _ _ _ _]
          tunnel: [w385 UI_State."Waiting for Exit (Log Stopped)" ("UI State") UI_State."Waiting for Stop (Log Stopped)" ("UI State") UI_State."Idle" ("UI State") UI_State."Idle" ("UI State")] -> w381
          tunnel: w380 -> [w384 w386 w388 w394 w400]
          tunnel: [w384 w386 w388 w393 w399] -> w374
          tunnel: w379 -> [_ _ _ w392 w398]
          frame Default {
          }
          frame "Waiting for Exit", "Waiting for Exit (Log Stopped)" {
          }
          frame "Waiting for Stop", "Waiting for Stop (Log Stopped)" {
          }
          frame "Waiting for Exit (Acq Stopped)" {
            # "If we are waiting to exit, and the acquisition has already stopped, then the \"Logging Stopped\" message indicates that it is time to exit."
            n130 = call-poly "Enqueue Message.vi"("Priority Message? (F)"=TRUE, "error in (no error)"=w394, "Message"="Exit", "Message Queue"=w392) -> ("error out"=w393:errorcluster)  [unwired: 6 in, 1 out]
          }
          frame "Waiting for Stop (Acq Stopped)" {
            # "If we are waiting to stop, and the acquisition has already stopped, then the \"Logging Stopped\" message indicates that it is time to stop."
            n131 = call-poly "Enqueue Message.vi"("error in (no error)"=w400, "Message Data"="Ready..." ("Message"), "Message"="Update Status", "Message Queue"=w398) -> ("error out"=w399:errorcluster)  [unwired: 6 in, 1 out]
          }
        }
        n132 = Unbundle By Name(w375) -> ("Centrifuge Module Config.Process Name"=w378:string)
        n133 = Concatenate Strings(w378, " Logging Stopped" ("text")) -> (w376:string)
        n134 = call "Write to Log File.vi"("error in"=w374, "text"=w376) -> ()  [unwired: 9 in, 1 out]
      }
      frame "Start" {
        # "Clear chart"
        # "Message Acquisition and Logging loops to start"
        # "Enable: Stop\nDisable: Start, Exit, Settings"
        # "Start - Enable/Disable buttons appropriately for an acquisition that has started, and update status display."
        n135 = Unbundle By Name(w410) -> ("Trigger Ref"=w418:refnum<vi>, "Stop Ref"=w419:refnum<vi>, "Start Ref"=w422:refnum<vi>, "Exit Ref"=w421:refnum<vi>, "Settings Ref"=w420:refnum<vi>, "Data Ref"=w412:refnum<vi>)
        n136 = property class="WFChart (strict)"(reference=w412, "History Data"=waveform(dbl)[][] []) -> ()  [unwired: 1 in, 2 out]
        n137 = Build Array(w422, w421, w420) -> (w425:refnum<vi>[])
        n138 = Build Array(w418, w419) -> (w424:refnum<vi>[])
        n139 = call "Set Enable State on Multiple Controls.vi"("Enable?"=TRUE, "Controls"=w424) -> ()  [unwired: 10 in]
        n140 = call "Set Enable State on Multiple Controls.vi"("Enable?"=FALSE, "Controls"=w425) -> ()  [unwired: 10 in]
        n141 = call-poly "Enqueue Message.vi"("error in (no error)"=w413, "Message"="Broadcast settings", "Message Queue"=w415) -> ("error out"=w416:errorcluster, "dup Message Queue"=w414:refnum<queue>)  [unwired: 7 in]
        n142 = in-place {
          in-place-border: w416 -> [w431]
          in-place-border: w414 -> [w430]
          in-place-border: [w429] -> w407
          n143 = in-place-cluster #3(w405) -> ("State"=w428:T10)
          n144 = case shown="Default" w428 {
            tunnel: [w433 w436] -> w432
            tunnel: w431 -> [w433 w435]
            tunnel: w430 -> [_ w434]
            frame "Measuring" {
            }
            frame Default {
              # "If it is not started yet, start"
              n145 = call-poly "Enqueue Message.vi"("error in (no error)"=w435, "Message"="Start Loops", "Message Queue"=w434) -> ("error out"=w436:errorcluster)  [unwired: 7 in, 1 out]
            }
          }
          n146 = Merge Errors(w432) -> (w429:errorcluster)
          n147 = in-place-cluster #3("State"=State_Enum."Measuring") -> (w404:T9)
        }
        n148 = Unbundle By Name(w404) -> ("Centrifuge Module Config.Process Name"=w403:string)
        n149 = Concatenate Strings(w403, " Start" ("text")) -> (w408:string)
        n150 = call "Write to Log File.vi"("error in"=w407, "text"=w408) -> ()  [unwired: 9 in, 1 out]
      }
      frame "Sequence Start" {
        # "Clear chart"
        # "Message Acquisition and Logging loops to start"
        # "Enable: Stop\nDisable: Start, Exit, Settings"
        # "Start - Enable/Disable buttons appropriately for an acquisition that has started, and update status display."
        n151 = Unbundle By Name(w450) -> ("Trigger Ref"=w457:refnum<vi>, "Stop Ref"=w458:refnum<vi>, "Start Ref"=w461:refnum<vi>, "Exit Ref"=w460:refnum<vi>, "Settings Ref"=w459:refnum<vi>, "Data Ref"=w452:refnum<vi>)
        n152 = property class="WFChart (strict)"(reference=w452, "History Data"=waveform(dbl)[][] []) -> ()  [unwired: 1 in, 2 out]
        n153 = Build Array(w461, w460, w459) -> (w464:refnum<vi>[])
        n154 = Build Array(w457, w458) -> (w463:refnum<vi>[])
        n155 = call-poly "Enqueue Message.vi"("error in (no error)"=w453, "Message"="Broadcast settings", "Message Queue"=w454) -> ("error out"=w438:errorcluster, "dup Message Queue"=w439:refnum<queue>)  [unwired: 7 in]
        n156 = call "Set Enable State on Multiple Controls.vi"("Enable?"=TRUE, "Controls"=w463) -> ()  [unwired: 10 in]
        n157 = call "Set Enable State on Multiple Controls.vi"("Enable?"=FALSE, "Controls"=w464) -> ()  [unwired: 10 in]
        n158 = case shown="False" w445 {
          selector: w445 -> [_ w471]
          tunnel: [TRUE w471] -> w447
          tunnel: w438 -> [w469 w472]
          tunnel: w439 -> [w467 _]
          tunnel: [w466 w472] -> w446
          frame False {
            # "Start the loop if it isn't started yet"
            n159 = call-poly "Enqueue Message.vi"("error in (no error)"=w469, "Message"="Start Loops", "Message Queue"=w467) -> ("error out"=w466:errorcluster)  [unwired: 7 in, 1 out]
          }
          frame True {
          }
        }
        n160 = Bundle By Name(cluster=w449, "State"=State_Enum."Measuring") -> (w440:T9)
        n161 = Merge Errors(w446) -> (w441:errorcluster)
        n162 = Unbundle By Name(w440) -> ("Centrifuge Module Config.Process Name"=w444:string)
        n163 = Concatenate Strings(w444, " Sequence Start" ("text")) -> (w442:string)
        n164 = call "Write to Log File.vi"("error in"=w441, "text"=w442) -> ()  [unwired: 9 in, 1 out]
      }
      frame "Start Loops" {
        # "I don't think we would have multiple loops but i'm leaving it here incase."
        # "Message Acquisition and Logging loops to start"
        # "Start - Enable/Disable buttons appropriately for an acquisition that has started, and update status display."
        n165 = Unbundle By Name(w475) -> ("Centrifuge Module Config.Process Name"=w476:string)
        n166 = Build Array(w479) -> (w477:refnum<queue>[])
        n167 = for {
          tunnel: w474 -> [w486]
          tunnel: [w485] -> w478 mode=indexing
          tunnel: w477 -> [w484] mode=indexing
          tunnel: w476 -> [w483]
          n168 = call-poly "Enqueue Message.vi"("error in (no error)"=w486, "Message Data"=w483, "Message"="Start", "Message Queue"=w484) -> ("error out"=w485:errorcluster)  [unwired: 6 in, 1 out]
        }
        n169 = Merge Errors(w474, w478) -> (w482:errorcluster)
      }
      frame "Start Log" {
        # "Message Acquisition and Logging loops to start"
        # "Start - Enable/Disable buttons appropriately for an acquisition that has started, and update status display."
        n170 = Unbundle By Name(w490) -> ("Centrifuge Module Config.Process Name"=w495:string)
        n171 = Build Array(w498) -> (w496:refnum<queue>[])
        n172 = for {
          tunnel: w489 -> [w504]
          tunnel: [w503] -> w497 mode=indexing
          tunnel: w496 -> [w502] mode=indexing
          tunnel: w495 -> [w501]
          n173 = call-poly "Enqueue Message.vi"("error in (no error)"=w504, "Message Data"=w501, "Message"="Start Log", "Message Queue"=w502) -> ("error out"=w503:errorcluster)  [unwired: 6 in, 1 out]
        }
        n174 = property class="VI"("Front Panel.Title"=w495) -> ()  [unwired: 2 in, 2 out]
        n175 = Merge Errors(w489, w497) -> (w491:errorcluster)
        n176 = Unbundle By Name(w490) -> ("Centrifuge Module Config.Process Name"=w494:string)
        n177 = Concatenate Strings(w494, " Start Log" ("text")) -> (w492:string)
        n178 = call "Write to Log File.vi"("error in"=w491, "text"=w492) -> ()  [unwired: 9 in, 1 out]
      }
      frame "Stop" {
        # "Pause the pump when we get a stop command"
        # "Enable: Start, Exit, Settings\nDisable: Stop"
        # "Stop - Enable/Disable buttons appropriately for an acquisition that has stopped, and update status display."
        n179 = Unbundle By Name(w534) -> ("Trigger Ref"=w525:refnum<vi>, "Stop Ref"=w526:refnum<vi>, "Start Ref"=w529:refnum<vi>, "Exit Ref"=w528:refnum<vi>, "Settings Ref"=w527:refnum<vi>)
        n180 = call-poly "Enqueue Message.vi"("error in (no error)"=w516, "Message"="Broadcast settings", "Message Queue"=w514) -> ("error out"=w515:errorcluster, "dup Message Queue"=w513:refnum<queue>)  [unwired: 7 in]
        n181 = Build Array(w529, w528, w527) -> (w532:refnum<vi>[])
        n182 = Build Array(w525, w526) -> (w531:refnum<vi>[])
        n183 = call-poly "Enqueue Message.vi"("error in (no error)"=w515, "Message Data"="Ready..." ("Ready..."), "Message"="Update Status", "Message Queue"=w513) -> ("error out"=w521:errorcluster)  [unwired: 6 in, 1 out]
        n184 = call "Set Enable State on Multiple Controls.vi"("Enable?"=FALSE, "Controls"=w531) -> ()  [unwired: 10 in]
        n185 = call "Set Enable State on Multiple Controls.vi"("Enable?"=TRUE, "Controls"=w532) -> ()  [unwired: 10 in]
        n186 = call-poly "Enqueue Message.vi"("error in (no error)"=w521, "Message"="Pause", "Message Queue"=w522) -> ("error out"=w519:errorcluster)  [unwired: 7 in, 1 out]
        n187 = case shown="Default" w523 {
          selector: w523 -> [_ w538]
          tunnel: [UI_State."Waiting for Stop" ("UI State") w538] -> w524
          frame Default {
          }
          frame "Waiting for Exit" {
          }
        }
        n188 = Merge Errors(w519) -> (w508:errorcluster)
        n189 = Bundle By Name(cluster=w518, "State"=State_Enum."Paused") -> (w507:T9)
        n190 = Unbundle By Name(w507) -> ("Centrifuge Module Config.Process Name"=w511:string)
        n191 = Concatenate Strings(w511, " Stop" ("text")) -> (w509:string)
        n192 = call "Write to Log File.vi"("error in"=w508, "text"=w509) -> ()  [unwired: 9 in, 1 out]
      }
      frame "Update Status" {
        # "Update Display - Convert the message data to a string to display in the Status indicator."
        n193 = Variant To Data(error in=w550, type="", Variant=w549) -> (data=w543:string, error out=w547:errorcluster)
        "Status" <- w543
        n194 = Unbundle By Name(w546) -> ("Trigger Ref"=w542:refnum<vi>, "Stop Ref"=w545:refnum<vi>)
        n195 = property class="Bool"(reference=w545) -> ("DisabledEnum"=w544:T14)  [unwired: 1 in, 2 out]
        n196 = case shown="\"Enabled\"" w544 {
          tunnel: w543 -> [w554 _]
          tunnel: w542 -> [w555 _]
          frame "Enabled" {
            # "Disable the Force Trigger only while we are logging."
            n197 = Build Array(w555) -> (w556:refnum<vi>[])
            n198 = Not Equal?(x="Logging" ("Logging"), y=w554) -> (x != y?=w552:bool)
            n199 = call "Set Enable State on Multiple Controls.vi"("Enable?"=w552, "Controls"=w556) -> ()  [unwired: 10 in]
          }
          frame "Disabled", Default {
          }
        }
        n200 = Merge Errors(w547) -> (w551:errorcluster)
      }
      frame Default {
        # "'Default' case only runs if there is a message that isn't defined in any of the other cases.  Output a programming error."
        n201 = Concatenate Strings("The invalid message string " ("string"), w559, " was received in Pump Module Main." ("string")) -> (w560:string)
        n202 = Bundle By Name(cluster=errorcluster {"status"=TRUE, "code"=1, "source"=""} ("error constant"), "source"=w560) -> (w558:errorcluster)
        n203 = Unbundle By Name(w564) -> ("Centrifuge Module Config.Process Name"=w567:string)
        n204 = Concatenate Strings(w567, " Incorrect Message Recieved: " ("text"), w559) -> (w565:string)
        n205 = call "Write to Log File.vi"("error in"=w558, "text"=w565) -> ()  [unwired: 9 in, 1 out]
      }
    }
    n206 = call "Error Handler - Message Handling Loop.vi"("error in (no error)"=w86, "Message Queue"=w84) -> ("dup error in"=w85:errorcluster, "dup Message Queue"=w70:refnum<queue>)  [unwired: 8 in]
  }
  "Sequence Started" <- w7
  n207 = while {
    tunnel: w22 -> [w581]
    tunnel: [w583] -> w29
    shift-right: [w582] -> w24
    shift-left: w27 -> [w587]
    tunnel: [w580] -> w16
    tunnel: w15 -> [w580]
    tunnel: w12 -> [w579]
    shift-right: [w576] -> _
    shift-left: w4 -> [w575]
    tunnel: [w571] -> w3
    tunnel: [w570] -> w2
    stop <- w586 stop-if-true
    # "Event Handling Loop"
    n208 = call "Dequeue Message.vi"("timeout in ms (-1)"=50, "Message Queue"=w579) -> ("error out"=w572:errorcluster, "Message Data"=w577:variant, "Message"=w578:string, "dup Message Queue"=w573:refnum<queue>)  [unwired: 6 in]
    n209 = Flush Queue(queue=w573, error in (no error)=w572) -> (queue out=w570:refnum<queue>)  [unwired: 2 out]
    n210 = case "Display Update" shown="\"Update\"" w578 {
      tunnel: w577 -> [_ w598]
      tunnel: [w588 w595] -> w576
      tunnel: w575 -> [w588 _]
      frame "False", Default {
      }
      frame "Update" {
        n211 = disable-structure shown="Disabled" {
          frame Disabled {
            n212 = property on="Speed" class="DigNum (strict)"("Visible"=TRUE) -> ()  [unwired: 2 in, 2 out]
          }
          frame Enabled {
          }
        }
        n213 = Variant To Data(type=T15 {"Centrifuge On?"=enum."Off", "Cycle Period"=500.0, "Current Centrifuge Speed"=0.0, "Output"=enum."Default"} ("FM Display"), Variant=w598) -> (data=w597:T15)  [unwired: 1 in, 1 out]
        n214 = property on="Speed" class="DigNum (strict)"("Caption.Text"="Speed" ("Label.Text")) -> ()  [unwired: 2 in, 2 out]
        n215 = Unbundle By Name(w597) -> ("Current Centrifuge Speed"=w591:dbl, "Centrifuge On?"=w596:enum16{"Off", "On", "Not Initialized"}, "Cycle Period"=w595:dbl)  [unwired: 1 out]
        n216 = property class="VI"() -> ("Front Panel.Title"=w589:string)  [unwired: 2 in, 2 out]
        n217 = Bundle By Name(cluster=cluster{"User Name":string, "Speed":dbl} {"User Name"="", "Speed"=0.0} ("Display Cluster"), "User Name"=w589, "Speed"=w591) -> (→"Display Cluster":cluster{"User Name":string, "Speed":dbl})
        n218 = case shown="\"Off\"" w596 {
          frame "Off" {
            n219 = local write "Ring"(u16 1 ("Ring")) -> ()
          }
          frame "On" {
            "Ring" <- u16 0 ("Ring")
          }
          frame "Not Initialized", Default {
            n220 = local write "Ring"(u16 2 ("Ring")) -> ()
          }
        }
      }
    }
    n221 = event shown="[1] Panel Resize" {
      selector: w587 -> [_ _ _ _ _ _ _]
      dyn-events: [_ _ _ _ _ _ _] -> w582
      timeout: w576 -> [_ _ _ _ _ _ _]
      tunnel: [_ _ _ _ TRUE ("Discard?") _ _] -> w586
      tunnel: w581 -> [w603 _ w617 w622 w626 w631 _]
      tunnel: [_ _ w615 w625 _ w633 _] -> w584
      tunnel: [w603 _ w616 w621 w626 w632 _] -> w585
      event Timeout {
        n222 = event-data() -> ()  [unwired: 1 in, 1 out]
      }
      event Panel Resize {
        n223 = event-data() -> ("NewBnds"=w611:T16)  [unwired: 1 in]
        n224 = local read "Original Width"() -> (w610:u32)
        n225 = call "Front End Resize.vi"("Starting Font"=16.2, "Area to Font Division"=1000.0, "Original Text Box Width"=64, "NewBnds"=w611, "Original Panel Width"=w610) -> ("New Text Box Width"=w605:u64, "New Font Size"=w604:dbl)  [unwired: 5 in]
        n226 = Add(x=w605, y=u64 35) -> (x+y=w606:u64)
        n227 = property on="Speed" class="DigNum (strict)"("NumText.FontSize"=w604) -> ()  [unwired: 2 in, 2 out]
        n228 = property on="Speed" class="DigNum (strict)"("Caption.FontSize"=w604) -> ()  [unwired: 2 in, 2 out]
        n229 = property on="Speed" class="DigNum (strict)"("Text Width"=w605) -> ()  [unwired: 2 in, 2 out]
        n230 = property on="User Name" class="Str"("Text.Width"=w606) -> ()  [unwired: 2 in, 2 out]
        n231 = Multiply(x=w605, y=0.4) -> (x*y=w609:dbl)
        n232 = property on="User Name" class="Str"("Text.Height"=w609) -> ()  [unwired: 2 in, 2 out]
        n233 = property on="User Name" class="Str"("Text.FontSize"=w604) -> ()  [unwired: 2 in, 2 out]
      }
      event Panel Close? {
        w618 = TRUE  # Priority Message
        n234 = event-data() -> ()  [unwired: 1 in, 1 out]
        n235 = call-poly "Enqueue Message.vi"("Priority Message? (F)"=w618, "Message"="Confirm Quit", "Message Queue"=w617) -> ("error out"=w615:errorcluster, "dup Message Queue"=w616:refnum<queue>)  [unwired: 7 in]
        n236 = event-data("Discard?"=TRUE) -> ()  [unwired: 1 in, 1 out]
      }
      event "Exit": Value Change {
        w623 = TRUE  # Priority Message
        # "The UI Message Loop handles sending the Exit message to other loops."
        n237 = event-data() -> ()  [unwired: 1 in, 1 out]
        n238 = call-poly "Enqueue Message.vi"("Priority Message? (F)"=w623, "Message"="Exit", "Message Queue"=w622) -> ("error out"=w625:errorcluster, "dup Message Queue"=w621:refnum<queue>)  [unwired: 7 in]
      }
      event User Event {
        # "The Message Handling Loop processed an \"Exit\" message, which fired this event to stop the Event Handling Loop."
        n239 = event-data() -> ()  [unwired: 1 in, 1 out]
        n240 = local write "Status"("Exit" ("Exit String")) -> ()
      }
      event "Settings Button": Mouse Down {
        n241 = event-data() -> ("PlatMods"=w630:T17)  [unwired: 1 in]
        n242 = Unbundle By Name(w630) -> ("Ctrl"=w629:bool)
        n243 = case shown="False" w629 {
          tunnel: [w637 w638] -> w633
          tunnel: [w636 w639] -> w632
          tunnel: w631 -> [w635 w639]
          frame False {
            n244 = call-poly "Enqueue Message.vi"("Message"="Launch Settings Dialog", "Message Queue"=w635) -> ("error out"=w637:errorcluster, "dup Message Queue"=w636:refnum<queue>)  [unwired: 8 in]
          }
          frame True {
            n245 = property class="VI"("BDWin.Open"=TRUE ("Block Diagram Window:Open")) -> (error out=w638:errorcluster)  [unwired: 2 in, 1 out]
          }
        }
      }
      event Key Down {
        n246 = event-data() -> ("ScanCode"=→"ScanCode":i16)  [unwired: 1 in]
      }
    }
    n247 = call "Error Handler - Event Handling Loop.vi"("error in (no error)"=w584, "Message Queue"=w585) -> ("dup error in"=w583:errorcluster, "dup Message Queue"=w571:refnum<queue>)  [unwired: 8 in]
  }
  n248 = call "Main Loop.vi"("error in (no error)"=w10, "Chart Notifier"=w17, "Message Queues"=w11) -> ("error out"=w18:errorcluster)  [unwired: 8 in]
  n249 = Unregister For Events(event registration refnum=w24, error in=w29) -> (error out=w25:errorcluster)
  n250 = Release Queue(queue=w3) -> ()  [unwired: 2 in, 3 out]
  n251 = Release Queue(queue=w2) -> ()  [unwired: 2 in, 3 out]
  n252 = Close Reference(reference=w16) -> ()  [unwired: 1 in, 1 out]
  n253 = Release Queue(queue=w1) -> ()  [unwired: 2 in, 3 out]
  n254 = Merge Errors(w25, w30, w10, w18) -> (w28:errorcluster)
  n255 = call "Destroy User Event - Stop.vi"("error in (no error)"=w28, "User Event - Stop"=w26) -> ()  [unwired: 9 in, 1 out]
